vi "Launch Configured Task.vi"(8 "error in (no error)":errorcluster, 10 "Task":refnum<class "Task.lvclass">, 11 "VolatusCore in":refnum<class "VolatusCore.lvclass">) -> (0 "error out":errorcluster, 3 "VolatusCore out":refnum<class "VolatusCore.lvclass">)   [LabVIEW 2020, in "Volatus.lvlib" / "VolatusCore.lvclass"]
uses:
  VolatusCore.lvclass
  VolatusConfig/Task/Task.lvclass
  VolatusCore.lvclass/VolatusCore.ctl
  Volatus.lvlib
  Task/Task.lvclass
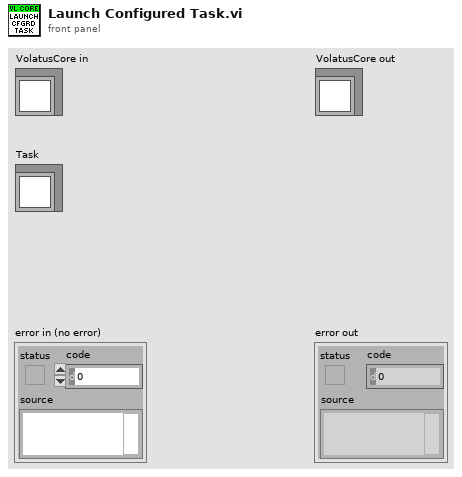
[diagram p1: front panel]
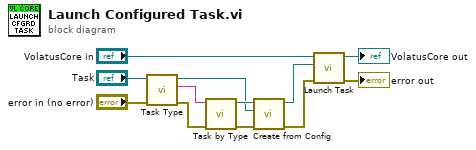
[diagram p0: block diagram]
diagram:
  n1 = call "Task Type.vi"("error in (no error)"="error in (no error)", "Task in"="Task") -> ("error out"=w9:errorcluster, "Task Type"=w8:string, "Task out"=w5:refnum<class "Task.lvclass">)  [unwired: 7 in]
  n2 = call "Task by Type.vi"("error in (no error)"=w9, "Task Type"=w8) -> ("error out"=w6:errorcluster, "Task"=w7:refnum<class "Task.lvclass">)  [unwired: 8 in]
  n3 = call "Create from Config.vi"("error in (no error)"=w6, "Config"=w5, "Task in"=w7) -> ("error out"=w2:errorcluster, "Task out"=w3:refnum<class "Task.lvclass">)  [unwired: 7 in]
  n4 = call "Launch Task.vi"("error in (no error)"=w2, "Task"=w3, "VolatusCore in"="VolatusCore in") -> ("error out"=→"error out":errorcluster, "VolatusCore out"=→"VolatusCore out":refnum<class "VolatusCore.lvclass">)  [unwired: 6 in, 1 out]
